vi "Keithley2100.constructor.vi"(0 "name":string, 2 "data in":string, 5 "error in (no error)":errorcluster) -> (14 "i ref out":refnum<vi>, 16 "data out":string, 19 "error out":errorcluster)   [LabVIEW 2014, in "Keithley2100.lvlib"]
doc: "This is the constructor of a class.\n\nLicense Agreement for this software:\n\nCopyright (C)\nGesellschaft für Schwerionenforschung, GSI\nPlanckstr. 1\n64291 Darmstadt\nGermany\n\nContact: D.Beck@gsi.de \n\nThis program is free software; you can redistribute it and/or modify it under the terms of the \nGNU General Public License as published by the Free Software Foundation; either version 2 of \nthe license, or (at your option) any later version.\n\nThis program is distributed in the hope that it will be useful, but WITHOUT ANY WARRANTY; \nwithout even the implied warranty of MERCHANTABILITY or FITNESS FOR A PARTICULAR PURPOSE. See the GNU General License for more details (http://www.gnu.org).\n\nGesellschaft für Schwerionenforschung, GSI\nPlanckstr. 1, 64291 Darmstadt, Germany\nFor all questions and ideas contact: M.Richter@gsi.de, H.Brand@gsi.de or D.Beck@gsi.de.\nLast update: 16-JUN-2004"
uses:
  Keithley2100.lvlib
  CS_Core/CSApplicationBaseClasses/DeviceBase/DeviceBase.myEventNames.ctl
  CS_Core/CSApplicationBaseClasses/DeviceBase/DeviceBase.lvlib
  CS_Core/CSSystem/CSSystemLib/CSSystemLib.lvlib
  CSlibraries-extern/DimLVEvent/LVDimInterface/LVDimInterface.lvlib
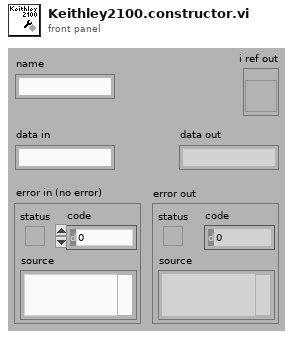
[diagram p1: front panel]
types:
  T1 = enum16{"SetAttribute", "GetAttribute", "CreateAttribute", "DestroyAttribute", "DestroyAllAtributes"}
  T2 = typedef "DeviceBase.lvlib/DeviceBase.myEventNames.ctl" = enum16{"lvmsg://Initialize", "lvmsg://Close", "lvmsg://Configure", "lvmsg://Reset", "lvmsg://IDQuery"}
  T3 = typedef "Keithley2100.lvlib/Keithley2100.i attribute.ctl" = cluster{"Custom Range":dbl, "Threshold Range":dbl, "VISA resource name":refnum<visa-resource-name>, "Auto Range":bool, "Digital Filter Readings":i32, "Digital Filter":u16, "NPLC":u16, "Display on":u16, "Resolution":u16, "Beaper enabled":bool, "MeasurementID":i32}
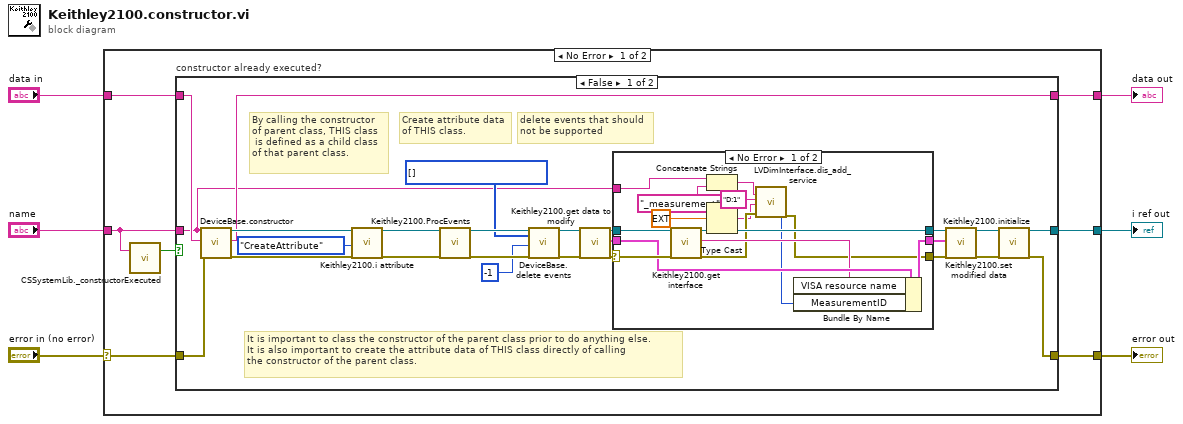
[diagram p0: block diagram]
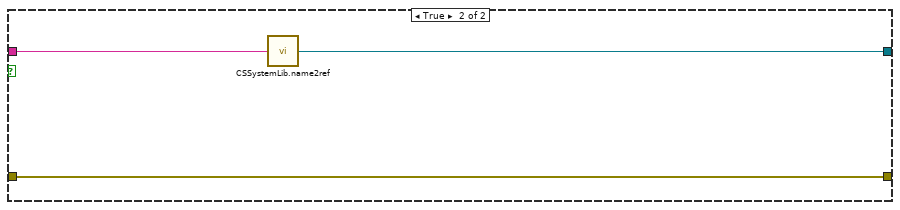
[diagram p3: hidden frame]
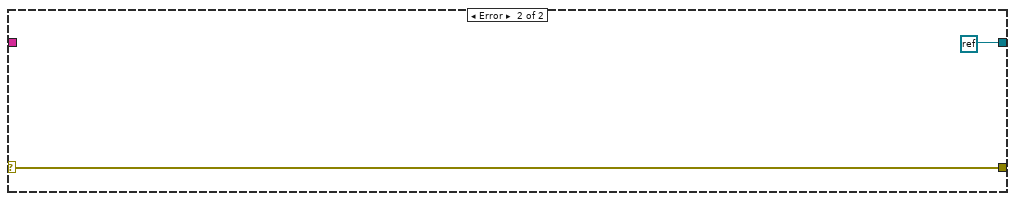
[diagram p4: hidden frame]
diagram:
  n1 = case shown="No Error" "error in (no error)" {
    selector: "error in (no error)" -> [w11 w60]
    tunnel: "name" -> [w10 _]
    tunnel: [w13 refnum<k0> refnum ("Not a Refnum Constant")] -> w5
    tunnel: [w12 w60] -> w4
    tunnel: "data in" -> [w8 _]
    tunnel: [w7 _] -> w1
    frame No Error {
      n2 = call "CSSystemLib._constructorExecuted.vi"("name"=w10) -> ("constructor executed?"=w9:bool)  [unwired: 18 in]
      n3 = case "constructor already executed?" shown="False" w9 {
        tunnel: w10 -> [w14 w59]
        tunnel: [w16 w58] -> w13
        tunnel: [w15 w57] -> w12
        tunnel: w11 -> [w33 w57]
        tunnel: w8 -> [w32 _]
        tunnel: [w27 _] -> w7
        frame False {
          w29 = T2[] [] items=["lvmsg://Initialize", "lvmsg://Close", "lvmsg://Configure", "lvmsg://Reset", "lvmsg://IDQuery"] ("events")
          # "delete events that should\nnot be supported"
          # "It is important to class the constructor of the parent class prior to do anything else.\nIt is also important to create the attribute data of THIS class directly of calling\nthe constructor of the parent class."
          # "Create attribute data\nof THIS class."
          # "By calling the constructor\nof parent class, THIS class\n is defined as a child class\nof that parent class."
          n4 = call "DeviceBase.constructor.vi"("name"=w14, "data in"=w32, "error in (no error)"=w33) -> ("i ref out"=w38:refnum<vi>, "data out"=w27:string, "error out"=w37:errorcluster)  [unwired: 14 in]
          n5 = call "Keithley2100.i attribute.vi"("VI Refnum"=w38, "Action"=T1."CreateAttribute", "error in (no error)"=w37) -> ("VI Refnum out"=w35:refnum<vi>, "error out"=w34:errorcluster)  [unwired: 14 in, 1 out]
          n6 = call "Keithley2100.ProcEvents.vi"("i ref in"=w35, "error in (no error)"=w34) -> ("i ref out"=w31:refnum<vi>, "error out"=w30:errorcluster)  [unwired: 16 in]
          n7 = call "DeviceBase.delete events.vi"("i ref in"=w31, "events"=w29, "ms timeout (10000)"=-1, "error in (no error)"=w30) -> ("i ref out"=w26:refnum<vi>, "error out"=w25:errorcluster)  [unwired: 13 in, 1 out]
          n8 = call "Keithley2100.get data to modify.vi"("i ref in"=w26, "error in (no error)"=w25) -> ("i ref out"=w23:refnum<vi>, "i attribute"=w22:T3, "error out"=w24:errorcluster)  [unwired: 14 in, 1 out]
          n9 = case shown="No Error" w24 {
            selector: w24 -> [w52 w55]
            tunnel: w23 -> [w53 w56]
            tunnel: w22 -> [w51 w54]
            tunnel: [w49 w56] -> w21
            tunnel: [w46 w55] -> w20
            tunnel: [w48 w54] -> w19
            tunnel: w14 -> [w44 _]
            frame No Error {
              n10 = call "Keithley2100.get interface.vi"("i ref in"=w53, "error in (no error)"=w52) -> ("i refout"=w49:refnum<vi>, "Interface"=w50:string, "error out"=w47:errorcluster)  [unwired: 15 in]
              n11 = Concatenate Strings(w44, "_measurement" ("string")) -> (w42:string)
              n12 = Type Cast(x=ext 0.0) -> (*(type *) &x=w40:string)  [unwired: 1 in]
              n13 = call "LVDimInterface.dis_add_service.vi"("serviceName"=w42, "typeDescriptor"="D:1", "data"=w40, "error in (no error)"=w47) -> ("my_serviceID"=w45:i32, "error out"=w46:errorcluster)  [unwired: 14 in]
              n14 = Bundle By Name(cluster=w51, "VISA resource name"=w50, "MeasurementID"=w45) -> (w48:T3)
            }
            frame Error {
            }
          }
          n15 = call "Keithley2100.set modified data.vi"("i ref in"=w21, "i attribute"=w19, "error in (no error)"=w20) -> ("i ref out"=w18:refnum<vi>, "error out"=w17:errorcluster)  [unwired: 15 in]
          n16 = call "Keithley2100.initialize.vi"("i ref in"=w18, "error in (no error)"=w17) -> ("i refout"=w16:refnum<vi>, "error out"=w15:errorcluster)  [unwired: 16 in]
        }
        frame True {
          n17 = call "CSSystemLib.name2ref.vi"("name"=w59) -> ("obj refnum"=w58:refnum<vi>)
        }
      }
    }
    frame Error {
    }
  }
  "i ref out" <- w5
  "error out" <- w4
  "data out" <- w1
